vi "AM Tx try 2.vi"() -> ()   [LabVIEW 2011]
uses:
  <vilib>/sound2/lvsound2.llb/Sound Data Format.ctl
  <vilib>/sound2/lvsound2.llb/Sampling Mode.ctl
  <vilib>/addons/Modulation/Analog/MT Modulate AM (DSB).vi
  <instrlib>/niUSRP/niUSRP Write Tx Data (CDB Cluster).vi
  <vilib>/sound2/lvsound2.llb/Sound Input Read (DBL).vi
  <vilib>/Waveform/WDTOps.llb/WDT Index Channel DBL.vi
  <vilib>/addons/Modulation/niAMT.lvlib
panel:
  out "Waveform Graph":waveform(dbl)(graph)
  in  "Use Wav?":bool
  in  "Wav File":path
  in  "modulation index":dbl=1.0 format="%.2f"
  in  "Sound Format":T1={"sample rate (S/s)"=22050.0, "number of channels"=2, "bits per sample"=16}
  out "coerced gain":dbl format="%#_6f"
  in  "device names":refnum<k15>="192.168.10.2"
  in  "active antenna":string="TX1"
  in  "Capture Time (sec)":i32=10000
  in  "timeout":dbl=10.0
  out "error out":errorcluster
  in  "stop":bool
  out "coerced carrier frequency":dbl=100000.0 format="%#_6p"
  out "coerced IQ rate":dbl=100000.0 format="%#_6p"
  in  "gain":dbl format="%#_6f"
  in  "carrier frequency":dbl=2000000000.0 format="%#_6p"
  in  "IQ rate":dbl=10000000.0 format="%#_6p"
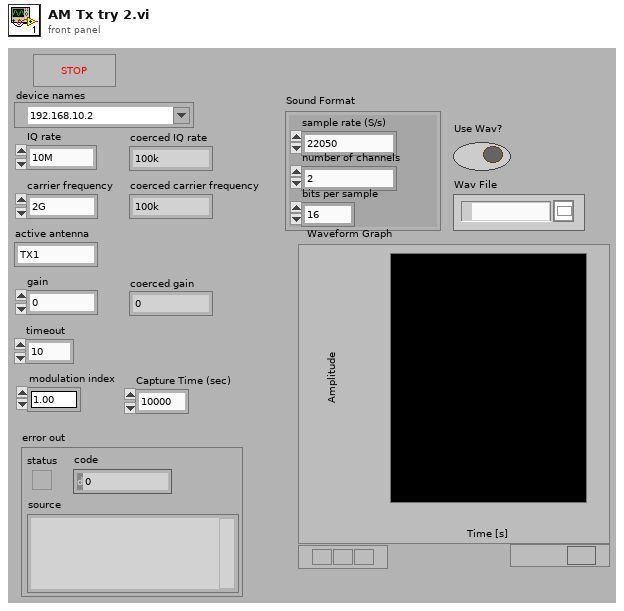
[diagram p1: front panel]
types:
  T1 = typedef "Sound Data Format.ctl" = cluster{"sample rate (S/s)":dbl, "number of channels":i32, "bits per sample":i32}
  T2 = typedef "Sampling Mode.ctl" = i32
  T3 = typedef "Semaphore RefNum" = refnum<k1>
  T4 = typedef "Sound Input Task ID.ctl" = u32
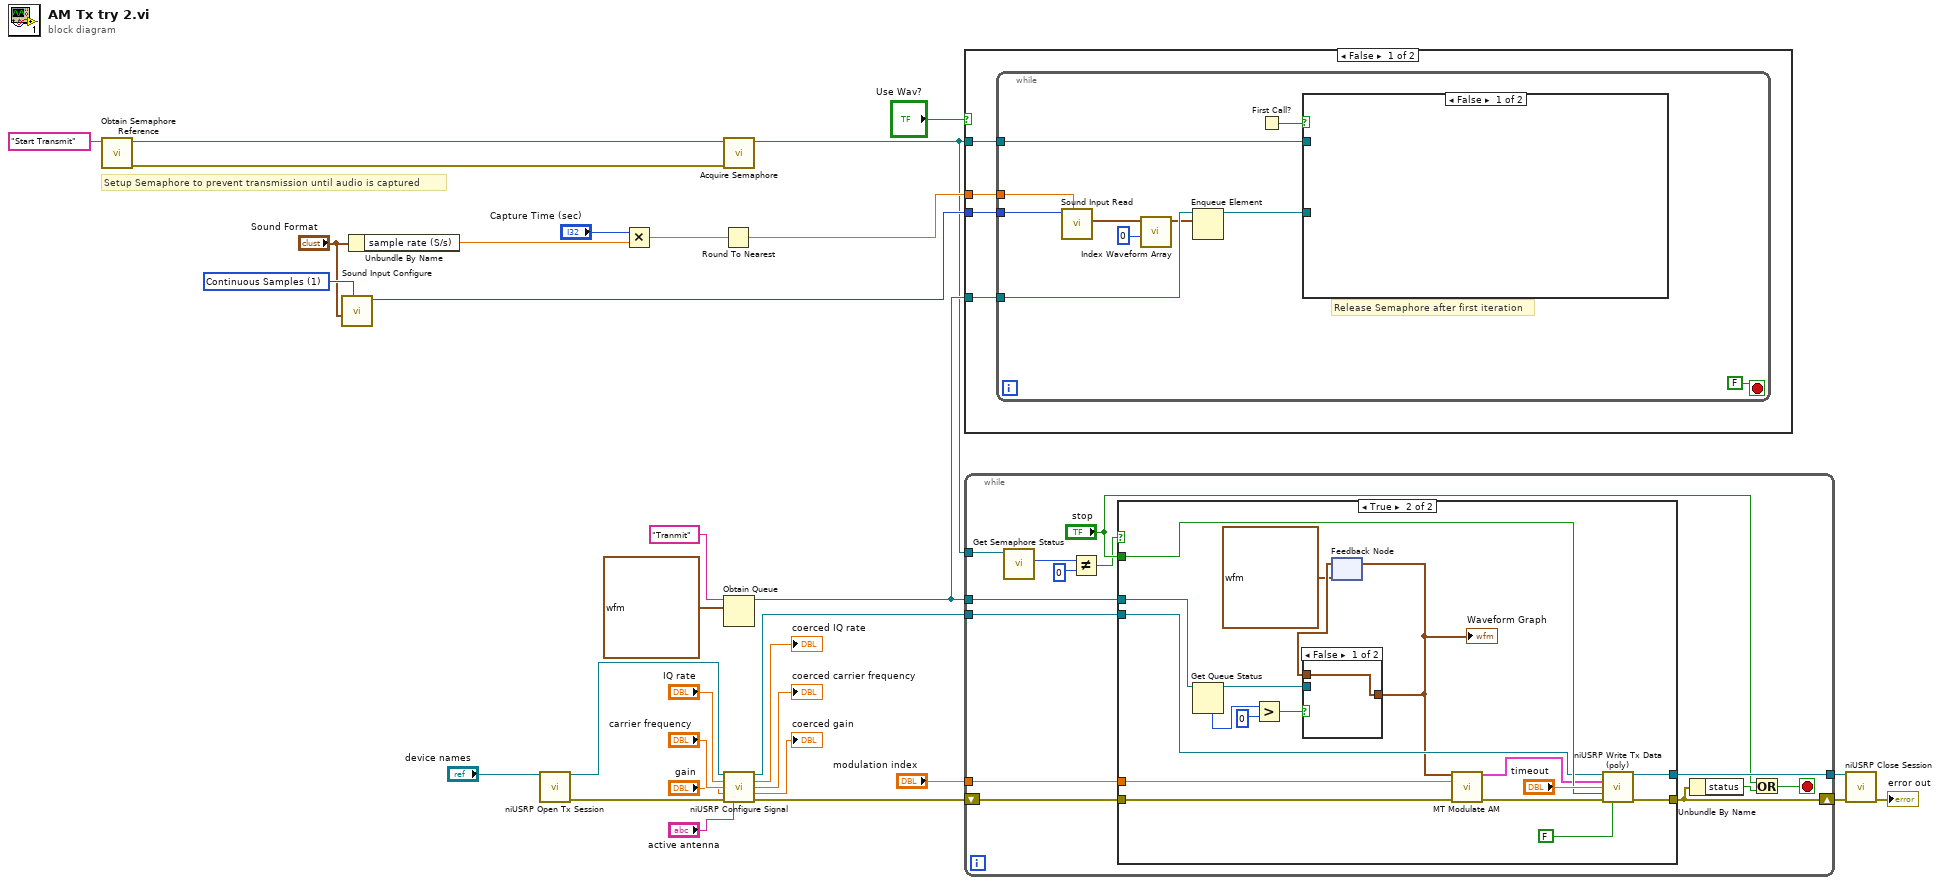
[diagram p0: block diagram]
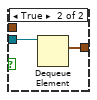
[diagram p3: hidden frame]
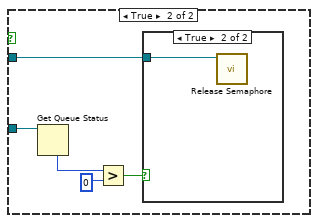
[diagram p4: hidden frame]
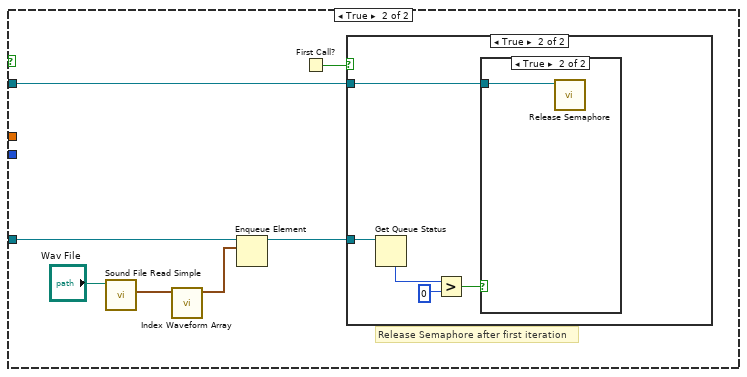
[diagram p6: hidden frame]
diagram:
  w23 = T2 1 items=["Finite Samples", "Continuous Samples"] ("sample mode")
  # "Setup Semaphore to prevent transmission until audio is captured"
  n1 = call <vilib>:"Obtain Semaphore Reference.vi"("name (unnamed)"="Start Transmit") -> ("error out"=w8:errorcluster, "semaphore"=w7:T3)  [unwired: 4 in, 1 out]
  n2 = call <vilib>:"Sound Input Configure.vi"("sample mode"=w23, "sound format"="Sound Format") -> ("task ID"=w13:T4)  [unwired: 8 in, 1 out]
  n3 = Unbundle By Name("Sound Format") -> ("sample rate (S/s)"=w15:dbl)
  n4 = call <instrlib>:"niUSRP Open Tx Session.vi"("device names"="device names") -> ("session handle out"=w31:refnum<k15>, "error out"=w29:errorcluster)  [unwired: 13 in]
  n5 = Multiply(x="Capture Time (sec)", y=w15) -> (x*y=w14:dbl)
  n6 = Round To Nearest(number=w14) -> (nearest integer value=w12:dbl)
  n7 = call <vilib>:"Acquire Semaphore.vi"("error in (no error)"=w8, "semaphore"=w7) -> ("semaphore out"=w1:T3)  [unwired: 3 in, 2 out]
  n8 = Obtain Queue(name (unnamed)="Tranmit", element data type=waveform(dbl) {"t0"=timestamp(0 s since 1904-01-01), "dt"=1.0, "Y"=[]} ("waveform")) -> (queue out=w6:refnum<queue>)  [unwired: 3 in, 2 out]
  n9 = call <instrlib>:"niUSRP Configure Signal.vi"("session handle"=w31, "IQ rate"="IQ rate", "carrier frequency"="carrier frequency", "gain"="gain", "error in (no error)"=w29, "active antenna"="active antenna") -> ("session handle out"=w19:refnum<k15>, "coerced IQ rate"=→"coerced IQ rate":dbl, "coerced carrier frequency"=→"coerced carrier frequency":dbl, "coerced gain"=→"coerced gain":dbl, "error out"=w20:errorcluster)  [unwired: 5 in]
  n10 = case shown="False" "Use Wav?" {
    tunnel: w13 -> [w35 _]
    tunnel: w12 -> [w34 _]
    tunnel: w1 -> [w33 w52]
    tunnel: w6 -> [w32 w53]
    frame False {
      n11 = while {
        tunnel: w35 -> [w45]
        tunnel: w34 -> [w44]
        tunnel: w32 -> [w43]
        tunnel: w33 -> [w37]
        stop <- FALSE stop-if-true
        # "Release Semaphore after first iteration"
        n12 = call-poly <vilib>:"Sound Input Read.vi"("number of samples/ch"=w44, "task ID"=w45) -> ("data"=w42:waveform(dbl)[])  [unwired: 7 in, 2 out]
        n13 = call-poly <vilib>:"Index Waveform Array.vi"("index"=0, "waveform array"=w42) -> ("waveform"=w40:waveform(dbl))  [unwired: 8 in, 1 out]
        n14 = Enqueue Element(queue=w43, element=w40) -> (queue out=w38:refnum<queue>)  [unwired: 2 in, 2 out]
        n15 = First Call?() -> (First Call?: T/F=w39:bool)
        n16 = case shown="False" w39 {
          tunnel: w38 -> [_ w50]
          tunnel: w37 -> [_ w47]
          frame False {
          }
          frame True {
            n17 = Get Queue Status(queue=w50) -> (# elements in queue=w49:i32)  [unwired: 2 in, 7 out]
            n18 = Greater?(x=w49, y=0) -> (0:w46:bool)
            n19 = case shown="True" w46 {
              tunnel: w47 -> [_ w51]
              frame False {
              }
              frame True {
                n20 = call <vilib>:"Release Semaphore.vi"("semaphore"=w51) -> ()  [unwired: 5 in, 2 out]
              }
            }
          }
        }
      }
    }
    frame True {
      # "Release Semaphore after first iteration"
      n21 = call <vilib>:"Sound File Read Simple.vi"("path"="Wav File") -> ("data"=w57:waveform(dbl)[])  [unwired: 7 in, 3 out]
      n22 = call-poly <vilib>:"Index Waveform Array.vi"("waveform array"=w57) -> ("waveform"=w54:waveform(dbl))  [unwired: 9 in, 1 out]
      n23 = Enqueue Element(queue=w53, element=w54) -> (queue out=w55:refnum<queue>)  [unwired: 2 in, 2 out]
      n24 = First Call?() -> (First Call?: T/F=w56:bool)
      n25 = case shown="True" w56 {
        tunnel: w55 -> [_ w63]
        tunnel: w52 -> [_ w60]
        frame False {
        }
        frame True {
          n26 = Get Queue Status(queue=w63) -> (# elements in queue=w62:i32)  [unwired: 2 in, 7 out]
          n27 = Greater?(x=w62, y=0) -> (0:w59:bool)
          n28 = case shown="True" w59 {
            tunnel: w60 -> [_ w64]
            frame False {
            }
            frame True {
              n29 = call <vilib>:"Release Semaphore.vi"("semaphore"=w64) -> ()  [unwired: 5 in, 2 out]
            }
          }
        }
      }
    }
  }
  n30 = while {
    tunnel: [w76] -> w3
    shift-right: [w75] -> w2
    shift-left: w20 -> [w71]
    tunnel: "modulation index" -> [w72]
    tunnel: w19 -> [w70]
    tunnel: w6 -> [w69]
    tunnel: w1 -> [w67]
    stop <- w77 stop-if-true
    n31 = call <vilib>:"Get Semaphore Status.vi"("semaphore"=w67) -> ("# available"=w68:i32)  [unwired: 5 in, 5 out]
    n32 = Not Equal?(x=w68, y=0) -> (x != y?=w66:bool)
    n33 = case shown="True" w66 {
      tunnel: [w79 w96] -> w76
      tunnel: [w78 w95] -> w75
      tunnel: "stop" -> [_ w94]
      tunnel: w72 -> [_ w91]
      tunnel: w71 -> [w78 w90]
      tunnel: w70 -> [w79 w88]
      tunnel: w69 -> [_ w87]
      frame False {
      }
      frame True {
        n34 = Get Queue Status(queue=w87) -> (queue out=w83:refnum<queue>, # elements in queue=w86:i32)  [unwired: 2 in, 6 out]
        n35 = Greater?(x=w86, y=0) -> (0:w84:bool)
        n36 = feedback #1(waveform(dbl) {"t0"=timestamp(0 s since 1904-01-01), "dt"=1.0, "Y"=[]} ("waveform")) -> (w82:waveform(dbl))
        n37 = case shown="False" w84 {
          tunnel: w83 -> [_ w100]
          tunnel: [w98 w99] -> w80
          tunnel: w82 -> [w98 _]
          frame False {
          }
          frame True {
            n38 = Dequeue Element(queue=w100) -> (element=w99:waveform(dbl))  [unwired: 2 in, 3 out]
          }
        }
        "Waveform Graph" <- w80
        n39 = feedback-in #1(w80) -> ()
        n40 = call-poly <vilib>:"MT Modulate AM.vi"("message signal"=w80, "modulation index"=w91, "error in (no error)"=w90) -> ("AM modulated waveform"=w93:cluster{"t0":dbl, "dt":dbl, "Y":cdb[]}, "error out"=w92:errorcluster)  [unwired: 11 in]
        n41 = call-poly <instrlib>:"niUSRP Write Tx Data (poly).vi"("session handle"=w88, "data"=w93, "timeout"="timeout", "end of data?"=w94, "error in (no error)"=w92, "use waveform dt for IQ rate?"=FALSE) -> ("session handle out"=w96:refnum<k15>, "error out"=w95:errorcluster)  [unwired: 8 in]
      }
    }
    n42 = Unbundle By Name(w75) -> ("status"=w74:bool)
    n43 = Or(x="stop", y=w74) -> (x .or. y?=w77:bool)
  }
  n44 = call <instrlib>:"niUSRP Close Session.vi"("session handle"=w3, "error in (no error)"=w2) -> ("error out"=→"error out":errorcluster)  [unwired: 13 in]
